vi "create_collection.vi"(0 "vector_weviate in":refnum<class "vector_weviate.lvclass">, 5 "collection_name":string, 7 "vector_size":u32, 9 "distance":string, 11 "error in (no error)":errorcluster) -> (4 "vector_weviate out":refnum<class "vector_weviate.lvclass">, 15 "error out":errorcluster)   [LabVIEW 2020, in "vector_weviate.lvclass"]
uses:
  vector_weviate.lvclass
  controls/collection data.ctl
  controls/collection properties.ctl
  vector_weviate.lvclass/vector_weviate.ctl
  <vilib>/httpClient/POSTBuffer.vi
  <vilib>/httpClient/LabVIEWHTTPClient.lvlib
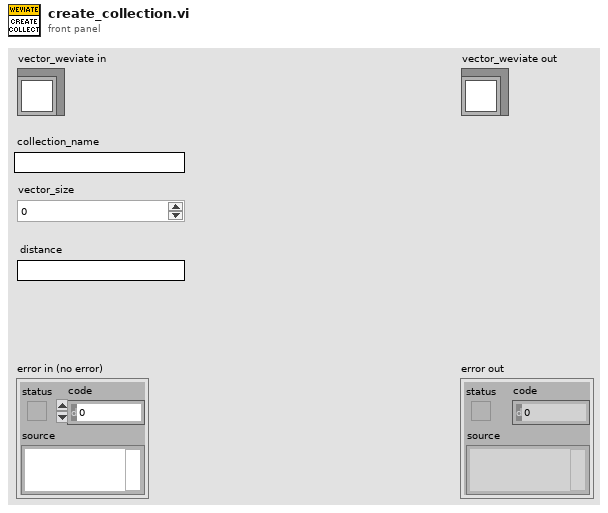
[diagram p1: front panel]
types:
  T1 = typedef "vector_weviate.lvclass/collection data.ctl" = cluster{"class":string, "properties":T2[], "distance":string}
  T2 = typedef "vector_weviate.lvclass/collection properties.ctl" = cluster{"name":string, "description":string, "data type":string}
  T3 = typedef "LabVIEWHTTPClient.lvlib/ClientHandle.ctl" = refnum<k1>
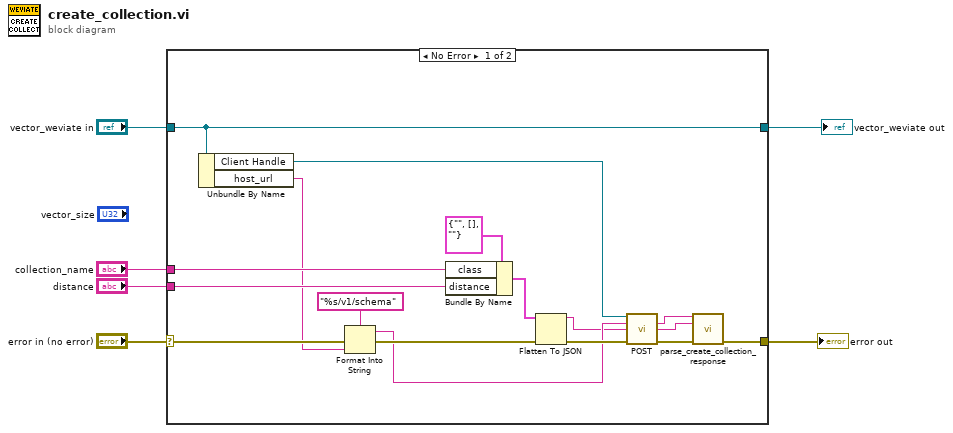
[diagram p0: block diagram]
diagram:
  n1 = case shown="No Error" "error in (no error)" {
    selector: "error in (no error)" -> [w18 w25]
    tunnel: "vector_weviate in" -> [w12 w24]
    tunnel: "collection_name" -> [w22 _]
    tunnel: "distance" -> [w21 _]
    tunnel: [w12 w24] -> w2
    tunnel: [w7 w25] -> w1
    frame No Error {
      n2 = Unbundle By Name(w12) -> ("Client Handle"=w19:T3, "host_url"=w11:string)
      n3 = Format Into String(format string="%s/v1/schema", error in=w18, w11) -> (resulting string=w14:string, error out=w16:errorcluster)  [unwired: 1 in]
      n4 = Bundle By Name(cluster=T1 {"class"="", "properties"=[], "distance"=""} ("collection data"), "class"=w22, "distance"=w21) -> (w20:T1)
      n5 = Flatten To JSON(anything=w20, error in (no error)=w16) -> (JSON string=w13:string, 11:w15:errorcluster)  [unwired: 1 in]
      n6 = call-poly <vilib>:"POST.vi"("client handle"=w19, "url"=w14, "buffer"=w13, "error in (no error)"=w15) -> ("headers"=w9:string, "body"=w8:string, "error out"=w10:errorcluster)  [unwired: 8 in, 1 out]
      n7 = call "parse_create_collection_response.vi"("headers"=w9, "body"=w8, "error in (no error)"=w10) -> ("error out"=w7:errorcluster)  [unwired: 12 in]
    }
    frame Error {
    }
  }
  "error out" <- w1
  "vector_weviate out" <- w2
